vi "G2CPU_ADD_Float.vi"(4 "Auto Release rhs (Enabled)":bool=TRUE, 6 "Auto Release lhs (Enabled)":bool=TRUE, 7 "batch":bool, 8 "error in (no error)":errorcluster, 9 "Array rhs":sgl, 11 "Array lhs":refnum<class "2D Array f32.lvclass">) -> (0 "error out":errorcluster, 2 "Array Result":refnum<class "2D Array f32.lvclass">)   [LabVIEW 2020]
doc: "Add 2 arrays with compatible sizes with each other.\nIf a scalar value is fed in, it will behave as an array of the exact same dimension count and size.\n\nWarning: When using scalar values, make sure the datatypes are the same.s"
uses:
  <vilib>/Natan Biesmans/G2CPU GPU and CPU HPC Toolkit/G2CPU Libraries/Arrays/2DArray/f32/2D Array f32.lvclass
  C:/Program Files/National Instruments/LabVIEW 2020/vi.lib/Natan Biesmans/G2CPU GPU and CPU HPC Toolkit/G2CPU Libraries/Arrays/Array/Array Prototype.lvclass
  20c5033d-e34b-4680-b71c-a1cccc2834c5.vi
  86f0bec7-6e21-4a72-bbfd-824d9a80339c.vi
  20c5033d-e34b-4680-b71c-a1cccc2834c5.vi/c3df215f-16d2-4e03-9745-9dd0f506ba18.vi
  20c5033d-e34b-4680-b71c-a1cccc2834c5.vi/c20e9e56-711a-4e3b-9a46-427845f2f903.vi
  20c5033d-e34b-4680-b71c-a1cccc2834c5.vi/80faa85e-9fb6-4da7-8f9b-44b1f9974ab2.vi
  20c5033d-e34b-4680-b71c-a1cccc2834c5.vi/730f6c57-5c0b-4ee9-b61e-75067b25222b.vi
  86f0bec7-6e21-4a72-bbfd-824d9a80339c.vi/2c12aba4-aacf-4d7a-adbe-039f6155a93e.vi
  86f0bec7-6e21-4a72-bbfd-824d9a80339c.vi/f38cccb2-46f6-49f0-a8d6-9da0c88ff6f3.vi
  86f0bec7-6e21-4a72-bbfd-824d9a80339c.vi/ac1e884d-1009-4464-9d84-e30609b15cc4.vi
  86f0bec7-6e21-4a72-bbfd-824d9a80339c.vi/b0150bb8-c0d1-462d-a788-37cf62685507.vi
  86f0bec7-6e21-4a72-bbfd-824d9a80339c.vi/12ac66bb-3c71-4165-9bea-8297abbfa9f1.vi
  20c5033d-e34b-4680-b71c-a1cccc2834c5.vi/c3df215f-16d2-4e03-9745-9dd0f506ba18.vi/601f24f8-2999-4f98-8030-64fd8876c127.vi
  20c5033d-e34b-4680-b71c-a1cccc2834c5.vi/c3df215f-16d2-4e03-9745-9dd0f506ba18.vi/e9745307-5113-4780-954c-71ccc9de0add.vi
  20c5033d-e34b-4680-b71c-a1cccc2834c5.vi/c20e9e56-711a-4e3b-9a46-427845f2f903.vi/c4afee3a-d58b-473f-ba2d-ee94fd2b49f4.vi
  20c5033d-e34b-4680-b71c-a1cccc2834c5.vi/80faa85e-9fb6-4da7-8f9b-44b1f9974ab2.vi/601f24f8-2999-4f98-8030-64fd8876c127.vi
  20c5033d-e34b-4680-b71c-a1cccc2834c5.vi/80faa85e-9fb6-4da7-8f9b-44b1f9974ab2.vi/e9745307-5113-4780-954c-71ccc9de0add.vi
  86f0bec7-6e21-4a72-bbfd-824d9a80339c.vi/ac1e884d-1009-4464-9d84-e30609b15cc4.vi/601f24f8-2999-4f98-8030-64fd8876c127.vi
  86f0bec7-6e21-4a72-bbfd-824d9a80339c.vi/ac1e884d-1009-4464-9d84-e30609b15cc4.vi/e9745307-5113-4780-954c-71ccc9de0add.vi
  86f0bec7-6e21-4a72-bbfd-824d9a80339c.vi/b0150bb8-c0d1-462d-a788-37cf62685507.vi/c5d3260c-dece-4fee-b11d-39452a92268b.vi
  86f0bec7-6e21-4a72-bbfd-824d9a80339c.vi/b0150bb8-c0d1-462d-a788-37cf62685507.vi/c5d3260c-dece-4fee-b11d-39452a92268b.vi/1a23f98f-393f-4176-8983-7f1ab824c539.vi
  <vilib>/Natan Biesmans/G2CPU GPU and CPU HPC Toolkit/G2CPU Libraries/Arrays/1DArray/f32/1D Array f32.lvclass
  <vilib>/Natan Biesmans/G2CPU GPU and CPU HPC Toolkit/ArrayFire Driver/VIs/Run as Multi Device.vi
  <vilib>/Natan Biesmans/G2CPU GPU and CPU HPC Toolkit/G2CPU Libraries/Manage Environment/Find AF DLL.vi
  <vilib>/Natan Biesmans/G2CPU GPU and CPU HPC Toolkit/ArrayFire Driver/subvi/Error Converter (ErrCode or Status).vi
  <vilib>/Natan Biesmans/G2CPU GPU and CPU HPC Toolkit/ArrayFire Driver/VIs/cast.vi
  <vilib>/Natan Biesmans/G2CPU GPU and CPU HPC Toolkit/G2CPU Libraries/Arrays/SubVI/Lock Arrays.vi
  <vilib>/Natan Biesmans/G2CPU GPU and CPU HPC Toolkit/G2CPU Libraries/Arrays/SubVI/is 2D.vi
  <vilib>/Natan Biesmans/G2CPU GPU and CPU HPC Toolkit/G2CPU Libraries/Arrays/Array/Array Prototype.lvclass
  <vilib>/Natan Biesmans/G2CPU GPU and CPU HPC Toolkit/G2CPU Libraries/Arrays/DataTypes/f32/f32.lvclass
  <vilib>/Natan Biesmans/G2CPU GPU and CPU HPC Toolkit/G2CPU Libraries/Arrays/2DArray/2D Array Prototype.lvclass
  <vilib>/Natan Biesmans/G2CPU GPU and CPU HPC Toolkit/ArrayFire Driver/AF.lvlib
  <vilib>/Natan Biesmans/G2CPU GPU and CPU HPC Toolkit/G2CPU Libraries/Garbage Collector/G2CPU GarbageCollectorAction.ctl
  <vilib>/Natan Biesmans/G2CPU GPU and CPU HPC Toolkit/G2CPU Libraries/Garbage Collector/Garbage Collector.lvlib
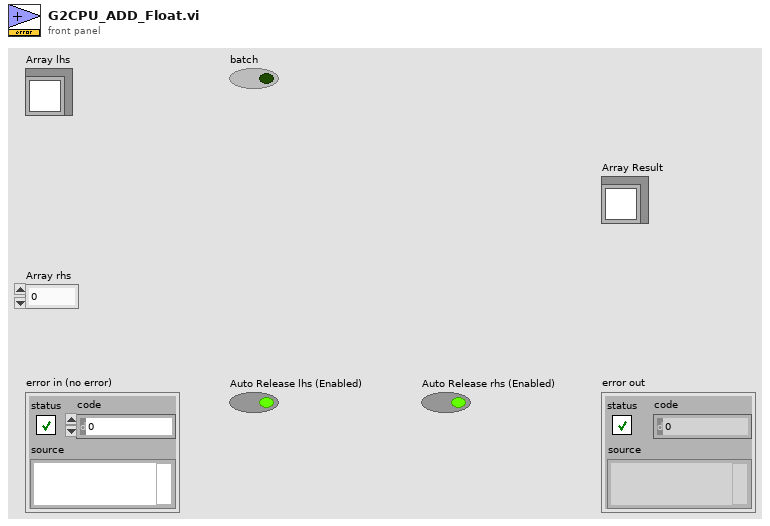
[diagram p1: front panel]
types:
  T1 = typedef "Garbage Collector.lvlib/G2CPU GarbageCollectorAction.ctl" = enum16{"Init", "Add", "Remove", "Flush"}
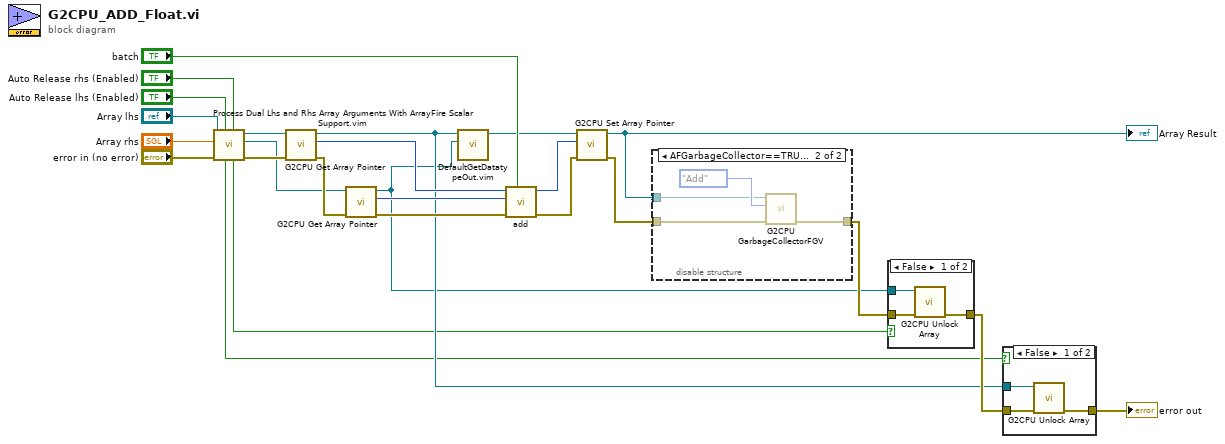
[diagram p0: block diagram]
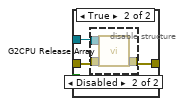
[diagram p2: hidden frame]
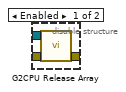
[diagram p3: hidden frame]
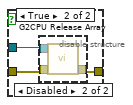
[diagram p4: hidden frame]
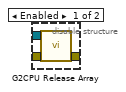
[diagram p5: hidden frame]
diagram:
  n1 = call "Process Dual Lhs and Rhs Array Arguments With ArrayFire Scalar Support.vim"("Auto Release rhs"="Auto Release rhs (Enabled)", "Auto Release lhs"="Auto Release lhs (Enabled)", "error in (no error)"="error in (no error)", "Array rhs"="Array rhs", "Array lhs"="Array lhs") -> ("error out"=w3:errorcluster, "Array rhs out"=w2:refnum<class "2D Array f32.lvclass">, "Array lhs out"=w1:refnum<class "2D Array f32.lvclass">, "Release rhs"=w4:bool, "Release lhs"=w5:bool)  [unwired: 2 in]
  n2 = call <vilib>:"G2CPU Get Array Pointer.vi"("error in (no error)"=w3, "Array in"=w1) -> ("error out"=w23:errorcluster, "Array Pointer"=w22:u64, "Array out"=w13:refnum<class "2D Array f32.lvclass">)  [unwired: 7 in]
  n3 = call <vilib>:"G2CPU Get Array Pointer.vi"("error in (no error)"=w23, "Array in"=w2) -> ("error out"=w24:errorcluster, "Array Pointer"=w21:u64, "Array out"=w11:refnum<class "2D Array f32.lvclass">)  [unwired: 7 in]
  n4 = call "DefaultGetDatatypeOut.vim"("Datatype In 2"=w11, "Datatype In 1"=w13) -> ("Datatype Out"=w12:refnum<class "2D Array f32.lvclass">)  [unwired: 9 in]
  n5 = call <vilib>:"add.vi"("batch"="batch", "error in (no error)"=w24, "Array Pointer rhs"=w21, "Array Pointer lhs"=w22) -> ("error out"=w19:errorcluster, "Array Pointer out"=w20:u64)  [unwired: 6 in]
  n6 = call <vilib>:"G2CPU Set Array Pointer.vi"("error in (no error)"=w19, "Array Pointer"=w20, "Array in"=w12) -> ("error out"=w18:errorcluster, "Array out"=w17:refnum<class "2D Array f32.lvclass">)  [unwired: 7 in]
  "Array Result" <- w17
  n7 = disable-structure shown="AFGarbageCollector==TRUE" {
    disable-tunnel: w17 -> [_ w29]
    disable-tunnel: w18 -> [w26 w28]
    disable-tunnel: [w26 w27] -> w14
    frame condition #0 (active) {
    }
    frame condition #1 {
      n8 = call <vilib>:"G2CPU GarbageCollectorFGV.vi"("error in (no error)"=w28, "Action"=G2CPU_GarbageCollectorAction."Add", "Array"=w29) -> ("error out"=w27:errorcluster)  [unwired: 7 in, 1 out]
    }
  }
  n9 = case shown="False" w4 {
    tunnel: w11 -> [w31 w35]
    tunnel: w14 -> [w33 w36]
    tunnel: [w32 w34] -> w16
    frame False {
      n10 = call <vilib>:"G2CPU Unlock Array.vi"("error in (no error)"=w33, "Array Prototype in"=w31) -> ("error out"=w32:errorcluster)  [unwired: 8 in, 1 out]
    }
    frame True {
      n11 = disable-structure shown="Disabled" {
        disable-tunnel: w36 -> [w39 w42]
        disable-tunnel: w35 -> [w38 w41]
        disable-tunnel: [w37 w40] -> w34
        frame Enabled {
          n12 = call <vilib>:"G2CPU Release Array.vi"("error in (no error)"=w39, "Array in"=w38) -> ("error out"=w37:errorcluster)  [unwired: 9 in]
        }
        frame Disabled {
          n13 = call <vilib>:"G2CPU Release Array.vi"("error in (no error)"=w42, "Array in"=w41) -> ("error out"=w40:errorcluster)  [unwired: 9 in]
        }
      }
    }
  }
  n14 = case shown="False" w5 {
    tunnel: w13 -> [w43 w47]
    tunnel: w16 -> [w45 w48]
    tunnel: [w44 w46] -> w15
    frame False {
      n15 = call <vilib>:"G2CPU Unlock Array.vi"("error in (no error)"=w45, "Array Prototype in"=w43) -> ("error out"=w44:errorcluster)  [unwired: 8 in, 1 out]
    }
    frame True {
      n16 = disable-structure shown="Disabled" {
        disable-tunnel: w48 -> [w51 w54]
        disable-tunnel: w47 -> [w50 w53]
        disable-tunnel: [w49 w52] -> w46
        frame Enabled {
          n17 = call <vilib>:"G2CPU Release Array.vi"("error in (no error)"=w51, "Array in"=w50) -> ("error out"=w49:errorcluster)  [unwired: 9 in]
        }
        frame Disabled {
          n18 = call <vilib>:"G2CPU Release Array.vi"("error in (no error)"=w54, "Array in"=w53) -> ("error out"=w52:errorcluster)  [unwired: 9 in]
        }
      }
    }
  }
  "error out" <- w15
